vi "poly_trim(s)_xwav(m).vi"(8 "Error in":errorcluster caption="Error in (no error)", 9 "end x (end)":dbl=inf, 10 "start x (start)":dbl=-inf, 11 "array of xwavs in":T1[](array[typedef])) -> (0 "Error out":errorcluster, 1 "actual end x index":i32, 2 "actual start x index":i32, 3 "array of xwavs out":T1[](array[typedef]))   [LabVIEW 2015, in "_xwav_polys.lvlib"]
uses:
  _xwav_polys.lvlib
  xwav.ctl
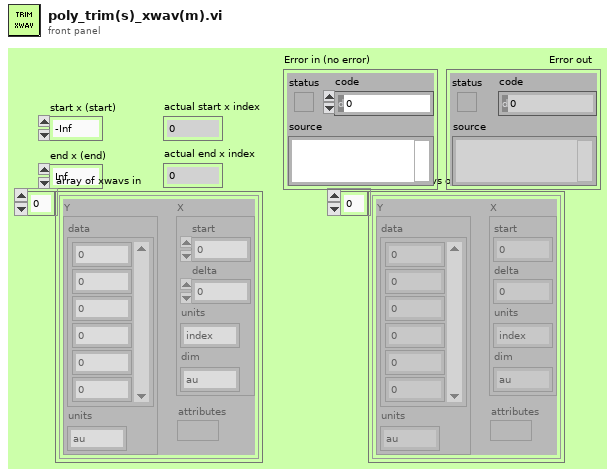
[diagram p1: front panel]
types:
  T1 = typedef "xwav.ctl" = cluster{"attributes":variant, "X":cluster{"start":dbl, "delta":dbl, "units":string, "dim":string}, "Y":cluster{"data":dbl[], "units":string}}
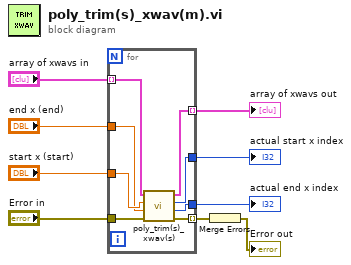
[diagram p0: block diagram]
diagram:
  n1 = for {
    tunnel: "end x (end)" -> [w10]
    tunnel: "start x (start)" -> [w11]
    tunnel: [w17] -> w7
    tunnel: [w16] -> w6
    tunnel: "array of xwavs in" -> [w15] mode=indexing
    tunnel: [w14] -> w4 mode=indexing
    tunnel: "Error in" -> [w13]
    tunnel: [w12] -> w2 mode=indexing
    n2 = call "poly_trim(s)_xwav(s).vi"("Error in"=w13, "end x (end)"=w10, "start x (start)"=w11, "xwave in"=w15) -> ("Error out"=w12:errorcluster, "actual end x index"=w16:i32, "actual start x index"=w17:i32, "xwave out"=w14:T1)  [unwired: 4 in]
  }
  "actual start x index" <- w7
  "actual end x index" <- w6
  "array of xwavs out" <- w4
  n3 = Merge Errors(w2) -> (→"Error out":errorcluster)
